vi "makePythonInstruction.vi"() -> ()   [LabVIEW 2020, in "Splitter.lvclass"]
uses:
  Splitter.lvclass
panel:
  out "Splitter en sortie":refnum<class "Splitter.lvclass">
  in  "Splitter.lvclass":refnum<class "Splitter.lvclass">
  out "error out 2":errorcluster caption="sortie d'erreur"
  in  "error in (no error) 2":errorcluster caption="entrée d'erreur (pas d'erreur)"
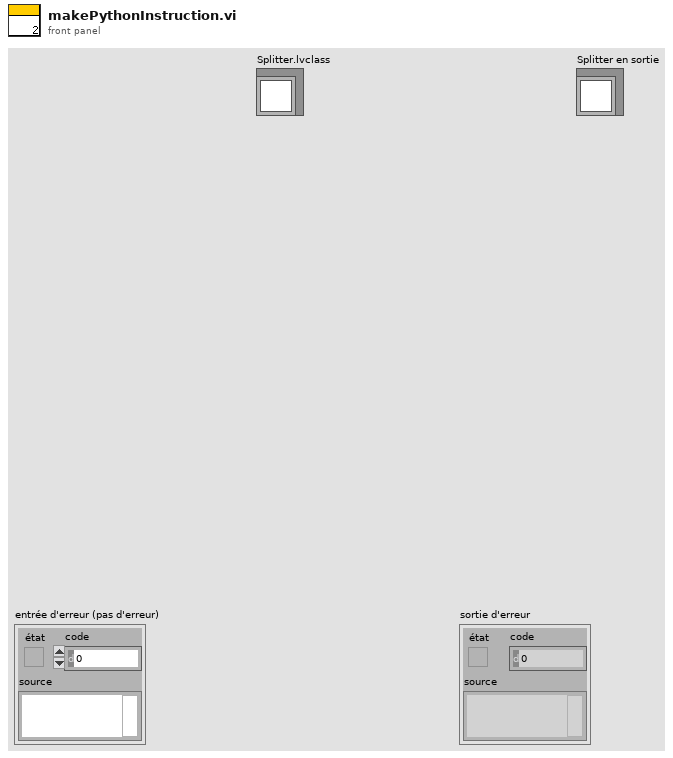
[diagram p1: front panel]
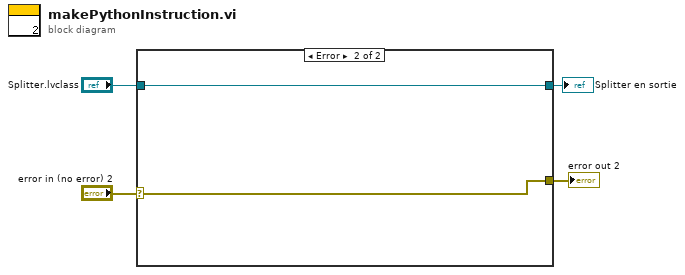
[diagram p0: block diagram]
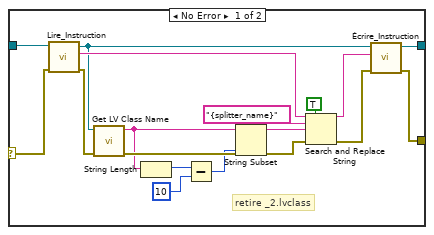
[diagram p2: hidden frame]
diagram:
  n1 = case shown="Error" "error in (no error) 2" {
    selector: "error in (no error) 2" -> [w11 w23]
    tunnel: [w7 w23] -> w3
    tunnel: "Splitter.lvclass" -> [w13 w22]
    tunnel: [w9 w22] -> w1
    frame No Error {
      # "retire _2.lvclass"
      n2 = call-dynamic "Lire_Instruction.vi"("error in (no error)"=w11, "Splitter en entrée"=w13) -> ("error out"=w10:errorcluster, "Instruction"=w12:string, "Splitter en sortie"=w5:refnum<class "Splitter.lvclass">)  [unwired: 7 in]
      n3 = call <vilib>:"Get LV Class Name.vi"("error in (no error)"=w10, "object"=w5) -> ("error out"=w20:errorcluster, "class name"=w18:string)  [unwired: 8 in]
      n4 = String Length(string=w18) -> (length=w17:i32)
      n5 = Subtract(x=w17, y=10) -> (x-y=w15:i32)
      n6 = String Subset(string=w18, length (rest)=w15) -> (substring=w19:string)  [unwired: 1 in]
      n7 = Search and Replace String(replace all?=TRUE ("tout remplacer ? (F)"), input string=w12, search string="{splitter_name}" ("chaîne recherchée"), replace string=w19, error in=w20) -> (result string=w6:string, error out=w8:errorcluster)  [unwired: 3 in, 2 out]
      n8 = call-dynamic "Écrire_Instruction.vi"("error in (no error)"=w8, "Instruction"=w6, "Splitter en entrée"=w5) -> ("error out"=w7:errorcluster, "Splitter en sortie"=w9:refnum<class "Splitter.lvclass">)  [unwired: 7 in]
    }
    frame Error {
    }
  }
  "error out 2" <- w3
  "Splitter en sortie" <- w1
